vi "Close.vi"(8 "error in":errorcluster, 11 "ExampleDevice in":refnum<class "ExampleDevice.lvclass">) -> (0 "error out":errorcluster, 3 "ExampleDevice out":refnum<class "ExampleDevice.lvclass">)   [LabVIEW 2023, in "ExampleDevice.lvclass"]
uses:
  ExampleDevice.lvclass
  ExampleDevice.lvclass/ExampleDevice.ctl
  Current Setpoint/Current Setpoint.lvclass
  Voltage Setpoint/Voltage Setpoint.lvclass
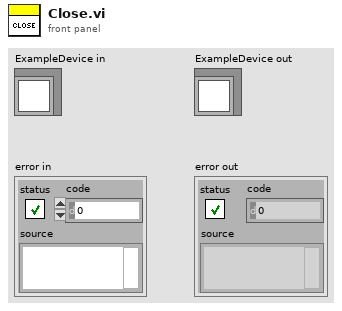
[diagram p1: front panel]
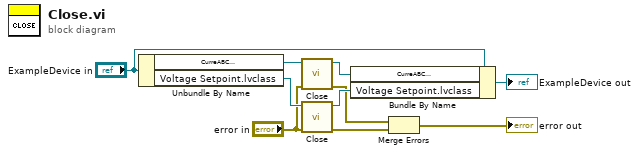
[diagram p0: block diagram]
diagram:
  n1 = Unbundle By Name("ExampleDevice in") -> ("CurreABC\n.lvclass"=w10:refnum<class "Current Setpoint.lvclass">, "Voltage Setpoint.lvclass"=w7:refnum<class "Voltage Setpoint.lvclass">)
  n2 = call-dynamic "Close.vi"("error in"="error in", "Setpoint in"=w10) -> ("error out"=w6:errorcluster, "Setpoint out"=w9:refnum<class "Current Setpoint.lvclass">)  [unwired: 8 in]
  n3 = call-dynamic "Close.vi"("error in"="error in", "Setpoint in"=w7) -> ("error out"=w5:errorcluster, "Setpoint out"=w8:refnum<class "Voltage Setpoint.lvclass">)  [unwired: 8 in]
  n4 = Bundle By Name(cluster="ExampleDevice in", "CurreABC\n.lvclass"=w9, "Voltage Setpoint.lvclass"=w8) -> (→"ExampleDevice out":refnum<class "ExampleDevice.lvclass">)
  n5 = Merge Errors(w6, w5) -> (→"error out":errorcluster)
